vi "force_sensor_model.vi"(10 "voltage_input":dbl) -> (2 "force_output":dbl)   [LabVIEW 2020]
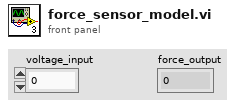
[diagram p1: front panel]
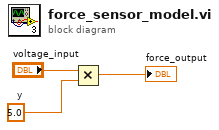
[diagram p0: block diagram]
diagram:
  w1 = 5.0  # y
  n1 = Multiply(x="voltage_input", y=w1) -> (x*y=→"force_output":dbl)
